vi "启动测量模式选择对话框.vi"(10 "启动选择":u16(ring) items=["水样测试", "标样核查", "零点核查", "加标回收", "平行样", "校零", "校标"], 11 "确定":bool) -> (3 "启动选择 3":u16(ring) items=["水样测量", "标样核查", "零点核查", "加标回收", "平行样", "校零", "校标", ""])   [LabVIEW 2016, in "斯坦道CODMn.lvlib"]
panel:
  in  "取消":bool
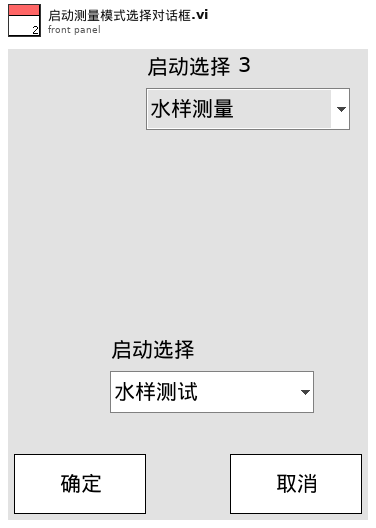
[diagram p1: front panel]
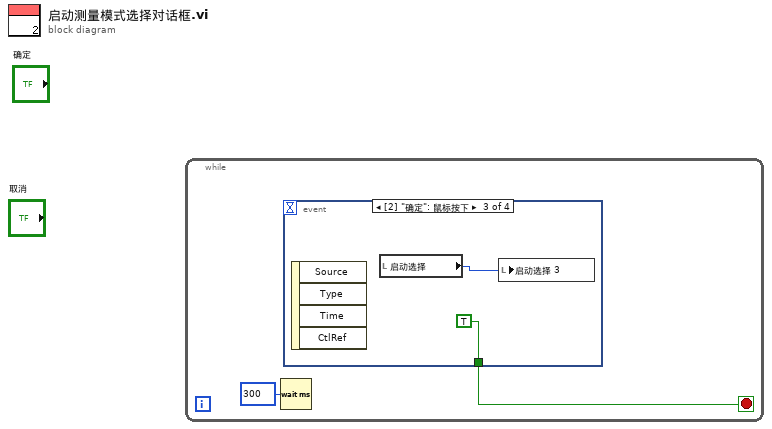
[diagram p0: block diagram]
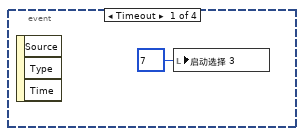
[diagram p2: hidden frame]
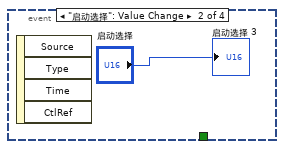
[diagram p3: hidden frame]
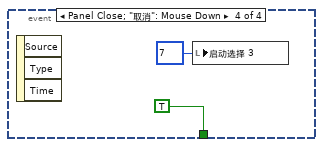
[diagram p4: hidden frame]
diagram:
  n1 = while {
    stop <- w2 stop-if-true
    n2 = Wait (ms)(milliseconds to wait=u32 300 ("等待时间（毫秒）")) -> ()  [unwired: 1 out]
    n3 = event shown="[2] \"确定\": 鼠标按下" {
      selector: _ -> [_ _ _ _]
      dyn-events: _ -> [_ _ _ _]
      timeout: _ -> [_ _ _ _]
      tunnel: [_ _ TRUE TRUE] -> w2
      event Timeout {
        w3 = u16 7 items=["水样测量", "标样核查", "零点核查", "加标回收", "平行样", "校零", "校标", ""] ("启动选择 3")
        n4 = event-data() -> ()  [unwired: 1 in, 3 out]
        n5 = local write "启动选择 3"(w3) -> ()
      }
      event "启动选择": Value Change {
        n6 = event-data() -> ()  [unwired: 1 in, 4 out]
        "启动选择 3" <- "启动选择"
      }
      event "确定": Mouse Down {
        n7 = event-data() -> ()  [unwired: 1 in, 4 out]
        n8 = local read "启动选择"() -> (w5:u16)
        n9 = local write "启动选择 3"(w5) -> ()
      }
      event Panel Close; "取消": Mouse Down {
        w7 = u16 7 items=["水样测量", "标样核查", "零点核查", "加标回收", "平行样", "校零", "校标", ""] ("启动选择 3")
        n10 = event-data() -> ()  [unwired: 1 in, 3 out]
        n11 = local write "启动选择 3"(w7) -> ()
      }
    }
  }
